vi "Merlin read freq.vi"(8 "error in (no error)":errorcluster, 10 "Freq":u32) -> (0 "error out":errorcluster)   [LabVIEW 2018]
uses:
  <vilib>/Instr/_visa.llb/VISA Configure Serial Port (Instr).vi
panel:
  in  "stop":bool
  out "Frequency":dbl
  out "Value":dbl
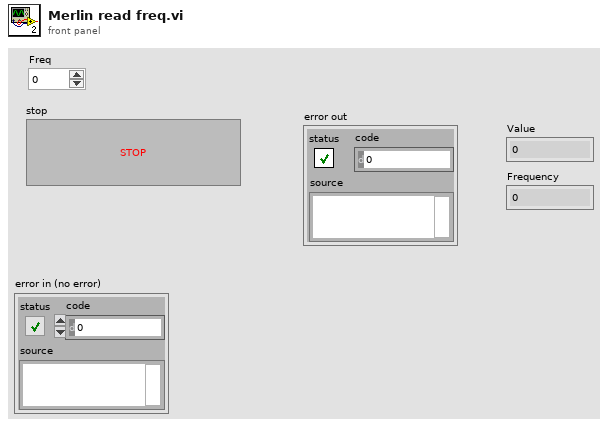
[diagram p1: front panel]
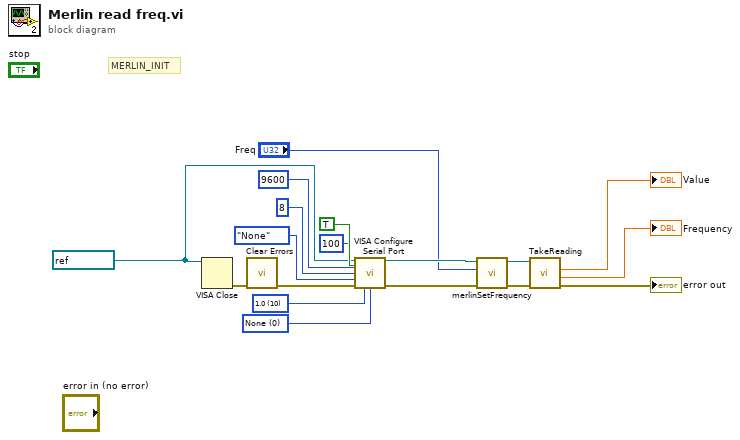
[diagram p0: block diagram]
diagram:
  w11 = refnum<visa-resource-name> "COM4" ("VISA resource name")
  w18 = u16 0 items=["None", "XON/XOFF", "RTS/CTS", "XON/XOFF & RTS/CTS", "DTR/DSR", "XON/XOFF & DTR/DSR"] ("flow control (0:none)")
  w17 = u16 10 items=["1.0"=10, "1.5"=15, "2.0"=20] ("stop bits (10: 1 bit)")
  # "MERLIN_INIT"
  n1 = VISA Close(VISA resource name=w11) -> (error out=w10:errorcluster)  [unwired: 1 in]
  n2 = call <vilib>:"Clear Errors.vi"("error in (no error)"=w10) -> ("error out"=w6:errorcluster)  [unwired: 5 in, 1 out]
  n3 = call-poly "VISA Configure Serial Port"("VISA resource name"=w11, "timeout (10sec)"=u32 100, "Enable Termination\nChar (T)"=TRUE ("Enable Termination\nChar (T)"), "baud rate (9600)"=u32 9600, "data bits (8)"=u16 8, "parity (0:none)"=enum16{"None", "Odd", "Even", "Mark", "Space"}."None", "error in (no error)"=w6, "stop bits (10: 1 bit)"=w17, "flow control (0:none)"=w18) -> ("VISA resource name out"=w8:refnum<visa-resource-name>, "error out"=w9:errorcluster)  [unwired: 5 in]
  n4 = call "merlinSetFrequency.vi"("error in"=w9, "Freq"="Freq", "Port"=w8) -> ("error out"=w4:errorcluster, "Port out"=w5:refnum<visa-resource-name>)  [unwired: 7 in]
  n5 = call "TakeReading.vi"("error in"=w4, "Port"=w5) -> ("error out"=→"error out":errorcluster, "Frequency"=→"Frequency":dbl, "Voltage(mV)"=→"Value":dbl)  [unwired: 6 in, 1 out]
